vi "Initialization VI for Wave Generator Memory.vi"() -> (0 "FXP Init Data Out":fxp<+/-,12,12>[](array[numeric]), 3 "Init Data Out":i64[](array[numeric]))   [LabVIEW 2014]
uses:
  <vilib>/Analysis/NI_AALPro.lvlib
  <vilib>/Analysis/NI_AALBase.lvlib
panel:
  out "Init Data Out Graph":i64[](graph)
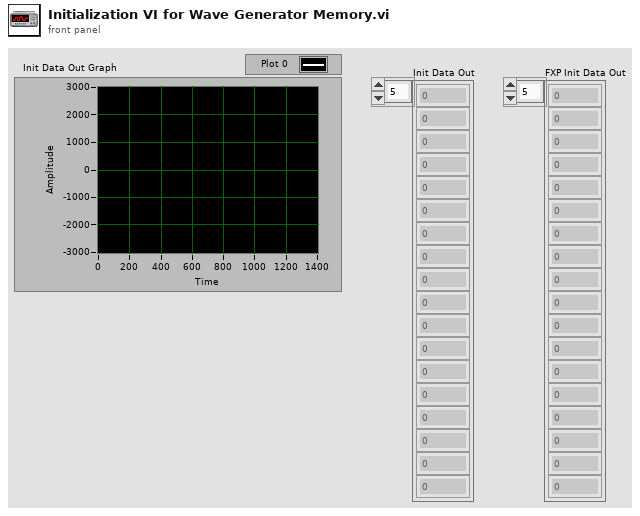
[diagram p1: front panel]
types:
  T1 = enum16{"sine", "cosine", "triangle", "square", "sawtooth", "increasing ramp", "decreasing ramp"}
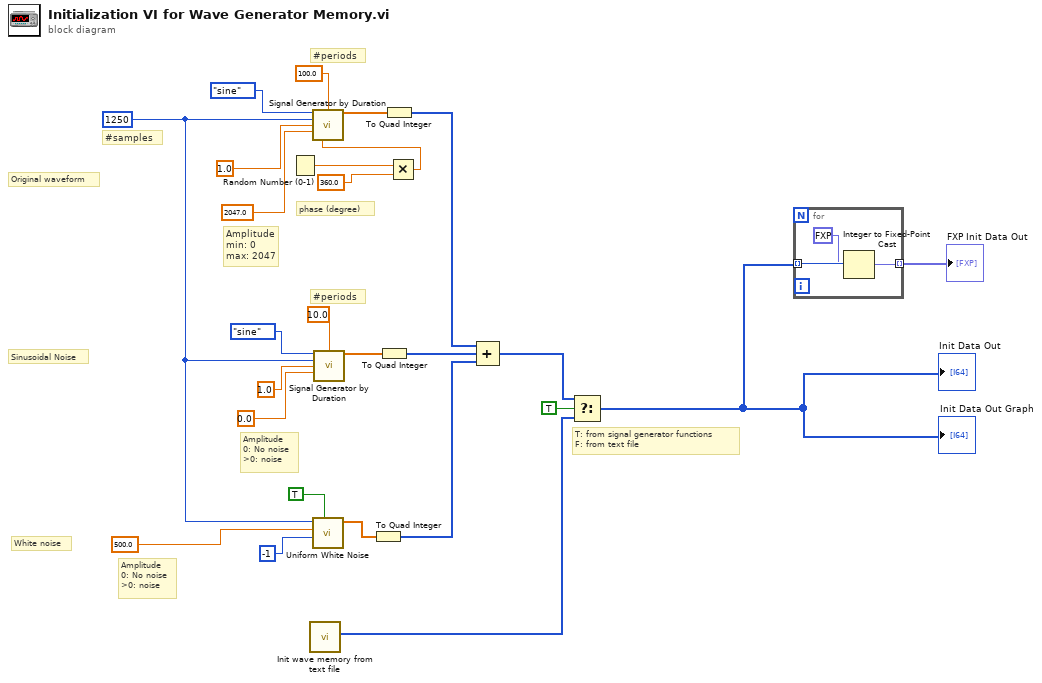
[diagram p0: block diagram]
diagram:
  w1 = 1250 ("# of samples")
  # "T: from signal generator functions\nF: from text file"
  # "Amplitude\n0: No noise\n>0: noise"
  # "Original waveform"
  # "Sinusoidal Noise"
  # "White noise"
  # "phase (degree)"
  # "#periods"
  # "Amplitude\n0: No noise\n>0: noise"
  # "#periods"
  # "Amplitude\nmin: 0\nmax: 2047"
  # "#samples"
  n1 = Random Number (0-1)() -> (number: 0 to 1=w7:dbl)
  n2 = call "Init wave memory from text file.vi"() -> ("Init Data Out"=w10:i64[])  [unwired: 11 in]
  n3 = call <vilib>:"Uniform White Noise.vi"("initialize?"=TRUE, "seed"=-1, "amplitude"=500.0, "samples"=w1) -> ("uniform white noise"=w2:dbl[])  [unwired: 6 in, 1 out]
  n4 = call <vilib>:"Signal Generator by Duration.vi"("signal type"=T1."sine", "duration"=10.0, "# of samples"=w1, "frequency"=1.0, "amplitude"=0.0) -> ("signal"=w23:dbl[])  [unwired: 7 in, 3 out]
  n5 = To Quad Integer(1:w2) -> (0:w16:i64[])
  n6 = To Quad Integer(1:w23) -> (0:w18:i64[])
  n7 = Multiply(x=w7, y=360.0) -> (x*y=w9:dbl)
  n8 = call <vilib>:"Signal Generator by Duration.vi"("signal type"=T1."sine", "duration"=100.0, "# of samples"=w1, "frequency"=1.0, "amplitude"=2047.0, "phase in"=w9) -> ("signal"=w3:dbl[])  [unwired: 6 in, 3 out]
  n9 = To Quad Integer(1:w3) -> (0:w15:i64[])
  n10 = Compound Arithmetic op=ADD(w15, w18, w16) -> (w12:i64[])
  n11 = Select(t=w12, s=TRUE, f=w10) -> (s? t:f=w13:i64[])
  "Init Data Out Graph" <- w13
  "Init Data Out" <- w13
  n12 = for {
    tunnel: w13 -> [w29] mode=indexing
    tunnel: [w27] -> w14 mode=indexing
    n13 = Integer to Fixed-Point Cast(fixed-point type=fxp<+/-,12,12> 0.0, integer=w29) -> (fixed-point=w27:fxp<+/-,12,12>)
  }
  "FXP Init Data Out" <- w14
